vi "calib.vi"() -> ()   [LabVIEW 2016]
uses:
  <vilib>/NXT/Block Support/NXT_OutputPort.ctl
  <vilib>/NXT/NXTIO Xnodes/NXTIONodeSubVIs/NXTMoveMotors.vi
  <vilib>/NXT/NXTIO Xnodes/NXTIONodeSubVIs/LEGOMotorStatus.vi
  <vilib>/NXT/NXTIO Xnodes/NXTIONodeSubVIs/NXTStopMotors.vi
  <vilib>/NXT/Subs/LVHSConnector.ctl
  <vilib>/NXT/NXTIO Xnodes/AddressXNode/NXTIOAddress.xnode
  <vilib>/NXT/NXTIO Xnodes/NXTIOXNode/NXTIO.xnode
  <vilib>/NXT/LegoClasses/BrickReference/BrickReference.lvclass
panel:
  in  "stop":bool
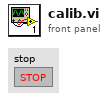
[diagram p1: front panel]
types:
  T1 = typedef "NXT_OutputPort.ctl" = u8
  T2 = cluster{"Output Port":T1, "Output Port 2":T1, "Output Port 3":T1}
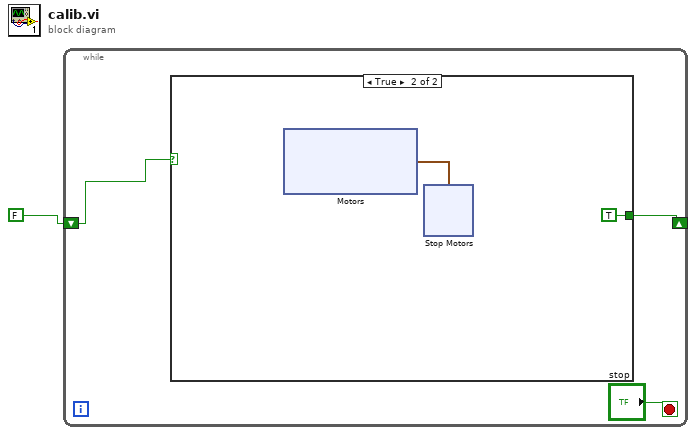
[diagram p0: block diagram]
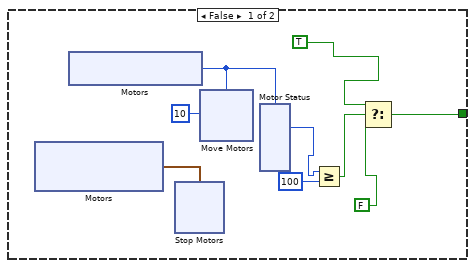
[diagram p2: hidden frame]
diagram:
  n1 = while {
    shift-right: [w3] -> _
    shift-left: FALSE -> [w2]
    stop <- "stop" stop-if-true
    n2 = case shown="True" w2 {
      tunnel: [w5 TRUE] -> w3
      frame False {
        n3 = xnode "Motors"() -> ("Motor"=w11:cluster{"Port":T1, "Port":T1})
        n4 = xnode "Motors"() -> ("Motor"=w12:T1)
        n5 = xnode "Stop Motors"("Motors"=w11) -> ()  [unwired: 1 in, 1 out]
        n6 = xnode "Move Motors"("Power/Speed 1"=i8 10, "Motors"=w12) -> ()  [unwired: 1 in, 1 out]
        n7 = xnode "Motor Status"("Motors"=w12) -> ("Position 1"=w10:i32)  [unwired: 1 in, 2 out]
        n8 = Greater Or Equal?(x=w10, y=100) -> (x >= y?=w8:bool)
        n9 = Select(t=TRUE, s=w8, f=FALSE) -> (s? t:f=w5:bool)
      }
      frame True {
        n10 = xnode "Motors"() -> ("Motor"=w37:cluster{"Port":T1, "Port":T1, "Port":T1})
        n11 = xnode "Stop Motors"("Motors"=w37) -> ()  [unwired: 1 in, 1 out]
      }
    }
  }
